vi "GetPropertyNative.vi"(8 "error in (no error)":errorcluster, 11 "reference in":refnum<class "G#MethodTemplates.lvclass">) -> (0 "error out":errorcluster, 2 "Numeric":dbl, 3 "reference out":refnum<class "G#MethodTemplates.lvclass">)   [LabVIEW 2017, in "G#MethodTemplates.lvclass"]
uses:
  <vilib>/addons/_AddQ/G#Templates/G#MethodTemplates/G#MethodTemplates.lvclass
  <vilib>/addons/_AddQ/G#Templates/G#MethodTemplates/G#MethodTemplates.lvclass/G#MethodTemplates.ctl
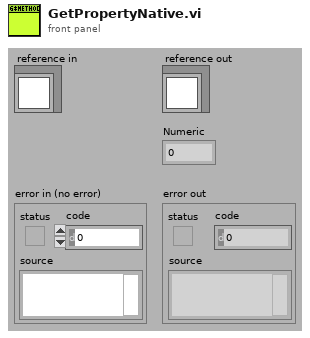
[diagram p1: front panel]
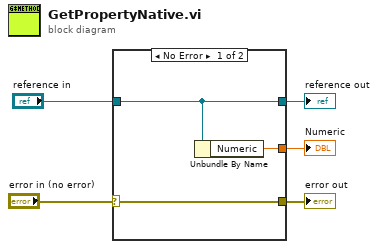
[diagram p0: block diagram]
diagram:
  n1 = case shown="No Error" "error in (no error)" {
    selector: "error in (no error)" -> [w6 w10]
    tunnel: [w6 w10] -> w4
    tunnel: [w8 w9] -> w2
    tunnel: "reference in" -> [w8 w9]
    tunnel: [w7 _] -> w1
    frame No Error {
      n2 = Unbundle By Name(w8) -> ("Numeric"=w7:dbl)
    }
    frame Error {
    }
  }
  "error out" <- w4
  "reference out" <- w2
  "Numeric" <- w1
